vi "SimpleSingleExponentialDecayMODEL.vi"(3 "output control":T1, 4 "data":T2, 5 "x":dbl[](array[numeric]), 6 "a":dbl[](array[numeric])) -> (0 "error out":errorcluster, 1 "f'(X,a)":dbl[][](array[numeric]), 2 "f(X, a)":dbl[](array[numeric]))   [LabVIEW 2016]
doc: "This template is the starting point for creating a model function to be passed to the Nonlinear Curve Fit.vi."
uses:
  <vilib>/gmath/NumericalOptimization/objective function data.ctl
  <vilib>/gmath/NumericalOptimization/LM_output select.ctl
  <vilib>/gmath/NI_Gmath.lvlib
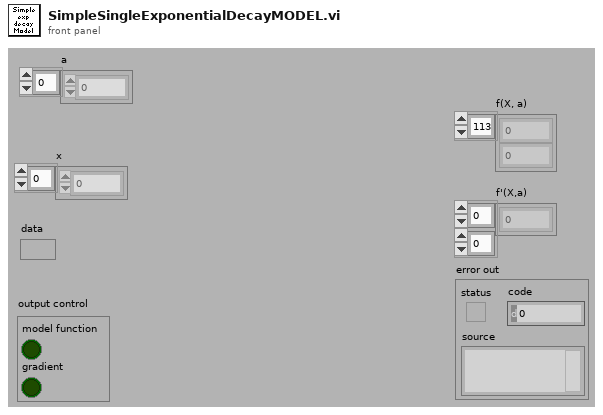
[diagram p1: front panel]
types:
  T1 = typedef "NI_Gmath.lvlib/LM_output select.ctl" = cluster{"model function":bool, "gradient":bool}
  T2 = typedef "NI_Gmath.lvlib/objective function data.ctl" = variant
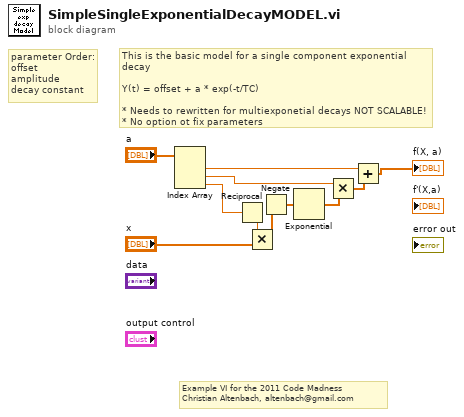
[diagram p0: block diagram]
diagram:
  # "This is the basic model for a single component exponential decay\n\nY(t) = offset + a * exp(-t/TC)\n\n* Needs to rewritten for multiexponetial decays NOT SCALABLE!\n* No option ot fix parameters"
  # "Example VI for the 2011 Code Madness\nChristian Altenbach, altenbach@gmail.com"
  # "parameter Order:\noffset\namplitude\ndecay constant"
  n1 = Index Array(array="a") -> (element #1=w3:dbl, element #2=w2:dbl, element #3=w1:dbl)  [unwired: 3 in]
  n2 = Reciprocal(x=w1) -> (1/x=w4:dbl)
  n3 = Multiply(x=w4, y="x") -> (x*y=w7:dbl[])
  n4 = Negate(x=w7) -> (-x=w5:dbl[])
  n5 = Exponential(1:w5) -> (0:w6:dbl[])
  n6 = Multiply(x=w2, y=w6) -> (x*y=w8:dbl[])
  n7 = Add(x=w3, y=w8) -> (x+y=→"f(X, a)":dbl[])
